vi "Set Axis Enable.vi"(4 "error in (no error)":errorcluster, 5 "Enable/Disable":bool=TRUE, 6 "Axis In":i16, 7 "Controller Reference":refnum<k7>) -> (0 "error out":errorcluster, 2 "Axis Out":i16, 3 "Controller Reference out":refnum<k7>)   [LabVIEW 2015]
doc: "Enables or Disables the selected Axis."
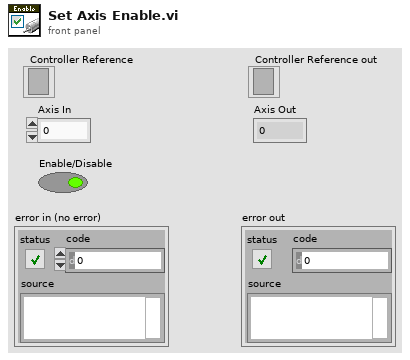
[diagram p1: front panel]
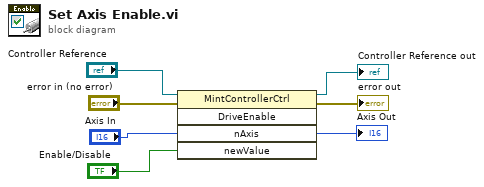
[diagram p0: block diagram]
diagram:
  n1 = invoke class="MintControllerCtrl" method="DriveEnable"(reference="Controller Reference", error in="error in (no error)", "nAxis"="Axis In", "newValue"="Enable/Disable") -> (reference out=→"Controller Reference out":refnum<k7>, error out=→"error out":errorcluster, "nAxis"=→"Axis Out":i16)  [unwired: 1 in, 2 out]
